vi "Oszi_KanalInfo.vi"(8 "Error In (No Error)":errorcluster, 10 "Oszi-Channel (1)":T1=1.0 min=1.0 max=4.0 step=1.0 format="%#_1g", 11 "VISA Name OZ In (OZ)":refnum<visa-resource-name>="USB0::0x0957::0x179B::MY54313507::INSTR") -> (0 "XINcrement":dbl, 1 "YREFerence":dbl, 2 "YORigin":dbl, 3 "YINcrement":dbl, 4 "Error Out":errorcluster, 5 "VISA Name OZ Out":refnum<visa-resource-name>="USB0::0x0957::0x179B::MY54313507::INSTR")   [LabVIEW 2016]
doc: "Gibt die entsprechenden Kanal-Infos des selektierten Kanals des Oszilloskops aus."
uses:
  Oszi_KanalInfo.ctl
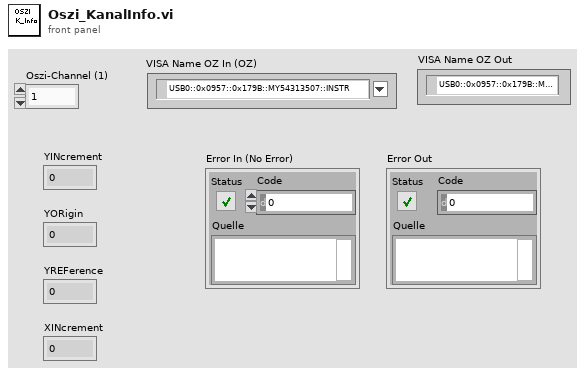
[diagram p1: front panel]
types:
  T1 = typedef "Oszi_KanalInfo.ctl" = dbl
  T2 = cluster{"[0]":refnum<visa-resource-name>, "[1]":refnum<visa-resource-name>, "[2]":refnum<visa-resource-name>, "[3]":refnum<visa-resource-name>, "[4]":refnum<visa-resource-name>, "[5]":refnum<visa-resource-name>, "[6]":refnum<visa-resource-name>, "[7]":refnum<visa-resource-name>, "[8]":refnum<visa-resource-name>}
  T3 = cluster{"[0]":string, "[1]":string, "[2]":string, "[3]":string, "[4]":string, "[5]":string, "[6]":string, "[7]":string, "[8]":string}
  T4 = cluster{"[0]":errorcluster, "[1]":errorcluster, "[2]":errorcluster, "[3]":errorcluster, "[4]":errorcluster, "[5]":errorcluster, "[6]":errorcluster, "[7]":errorcluster, "[8]":errorcluster}
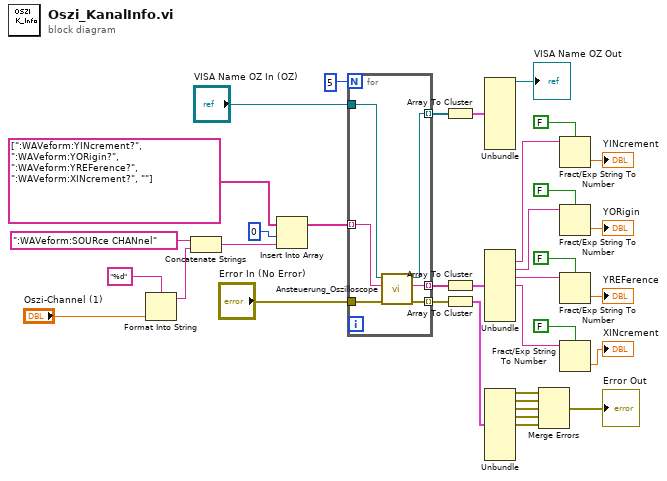
[diagram p0: block diagram]
diagram:
  n1 = Format Into String(format string="%d", "Oszi-Channel (1)") -> (resulting string=w4:string)  [unwired: 2 in, 1 out]
  n2 = Concatenate Strings(":WAVeform:SOURce CHANnel" ("string"), w4) -> (w2:string)
  n3 = Insert Into Array(array=string[] [":WAVeform:YINcrement?", ":WAVeform:YORigin?", ":WAVeform:YREFerence?", ":WAVeform:XINcrement?", ""], index=0, new element=w2) -> (w1:string[])
  n4 = for {
    N: 5 -> [_]
    tunnel: [w42] -> w23 mode=indexing
    tunnel: w1 -> [w41] mode=indexing
    tunnel: [w40] -> w31 mode=indexing
    tunnel: "Error In (No Error)" -> [w39]
    tunnel: "VISA Name OZ In (OZ)" -> [w38]
    tunnel: [w37] -> w22 mode=indexing
    n5 = call "Ansteuerung_Oszilloscope.vi"("Error_in"=w39, "Eingangs-String"=w41, "VISA Name OZ in(OZ)"=w38) -> ("Error_out"=w42:errorcluster, "Ausgangs-String"=w40:string, "VISA Name OZ out"=w37:refnum<visa-resource-name>)  [unwired: 6 in]
  }
  n6 = Array To Cluster(array=w22) -> (cluster=w21:T2)
  n7 = Array To Cluster(array=w31) -> (cluster=w32:T3)
  n8 = Array To Cluster(array=w23) -> (cluster=w20:T4)
  n9 = Unbundle(w21) -> ("[0]"=→"VISA Name OZ Out":refnum<visa-resource-name>)  [unwired: 8 out]
  n10 = Unbundle(w32) -> ("[1]"=w12:string, "[2]"=w11:string, "[3]"=w10:string, "[4]"=w9:string)  [unwired: 5 out]
  n11 = Unbundle(w20) -> ("[0]"=w19:errorcluster, "[1]"=w18:errorcluster, "[2]"=w17:errorcluster, "[3]"=w16:errorcluster, "[4]"=w13:errorcluster)  [unwired: 4 out]
  n12 = Merge Errors(w19, w18, w17, w16, w13) -> (→"Error Out":errorcluster)
  n13 = Fract/Exp String To Number(use system decimal point (T)=FALSE, string=w12) -> (number=→"YINcrement":dbl)  [unwired: 2 in, 1 out]
  n14 = Fract/Exp String To Number(use system decimal point (T)=FALSE, string=w11) -> (number=→"YORigin":dbl)  [unwired: 2 in, 1 out]
  n15 = Fract/Exp String To Number(use system decimal point (T)=FALSE, string=w10) -> (number=→"YREFerence":dbl)  [unwired: 2 in, 1 out]
  n16 = Fract/Exp String To Number(use system decimal point (T)=FALSE, string=w9) -> (number=→"XINcrement":dbl)  [unwired: 2 in, 1 out]
